vi "Teardown.vi"(11 "jettl Queue Actor in":refnum<class "jettl Queue Actor.lvclass">) -> (3 "jettl Queue Actor out":refnum<class "jettl Queue Actor.lvclass">)   [LabVIEW 2021, in "jettl Queue Actor.lvlib" / "jettl Queue Actor.lvclass"]
uses:
  jettl Queue Actor.lvclass
  State/Teardown State/Teardown State.lvclass
  C:/git/jettl/src/jettl/jettl Queue Actor/State/State/State.lvclass
  jettl Queue Actor.lvclass/jettl Queue Actor.ctl
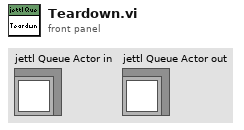
[diagram p1: front panel]
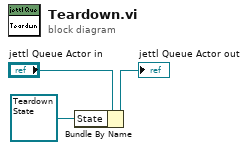
[diagram p0: block diagram]
diagram:
  n1 = Bundle By Name(cluster="jettl Queue Actor in", "State"=refnum<class "Teardown State.lvclass"> refnum ("LVCAM.lvlib:Destroying Self Actor State.lvclass")) -> (→"jettl Queue Actor out":refnum<class "jettl Queue Actor.lvclass">)
